vi "Delete from Array (Single).vi"(8 "index":i32, 11 "JSON Value in":refnum<class "JSON Value.lvclass">) -> (1 "JSON Value out":refnum<class "JSON Value.lvclass">, 3 "JSON Value out":refnum<class "JSON Value.lvclass">)   [LabVIEW 2016, in "JSON Value.lvclass"]
doc: "Deletes an element or subarray from a JSON array of length elements starting at index. Returns the edited array in array w/ subset deleted and the deleted element or subarray in deleted portion."
uses:
  JSON Value.lvclass
  JSON Value.lvclass/JSON Value.ctl
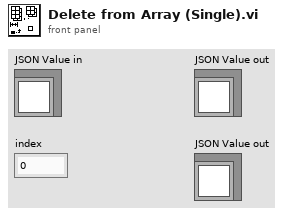
[diagram p1: front panel]
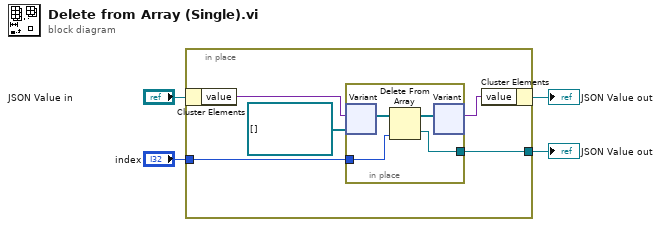
[diagram p0: block diagram]
diagram:
  n1 = in-place {
    in-place-border: "index" -> [w9]
    in-place-border: [w8] -> w1
    n2 = in-place-cluster #1("JSON Value in") -> ("value"=w7:variant)
    n3 = in-place {
      in-place-border: w9 -> [w13]
      in-place-border: [w12] -> w8
      n4 = in-place-variant #2(w7, refnum<class "JSON Value.lvclass">[] [] ("LVJSON.lvlib:JSON Array In")) -> (w11:refnum<class "JSON Value.lvclass">[])  [unwired: 1 out]
      n5 = Delete From Array(array=w11, index=w13) -> (deleted portion=w12:refnum<class "JSON Value.lvclass">, array with subset deleted=w10:refnum<class "JSON Value.lvclass">[])  [unwired: 1 in]
      n6 = in-place-variant #2(w10) -> (w5:variant)  [unwired: 1 out]
    }
    n7 = in-place-cluster #1("value"=w5) -> (→"JSON Value out":refnum<class "JSON Value.lvclass">)
  }
  "JSON Value out" <- w1
